vi "Intialize Sessions - 1Sess.vi"(6 "initialize and close session behavior":T1, 7 "option string":string, 8 "error in":errorcluster, 11 "session reservation in":refnum<class "Session Reservation.lvclass">) -> (0 "error out":errorcluster, 2 "session":refnum<class "Session Factory.lvclass">, 3 "session reservation out":refnum<class "Session Reservation.lvclass">)   [LabVIEW 2021, in "NI Session Management niSE.lvlib"]
uses:
  NI Session Management niSE.lvlib
  <vilib>/Plug-In SDKs/Clients/Session Management V1/Session Reservation/Session Reservation.lvclass
  <vilib>/Plug-In SDKs/Clients/Session Management V1/Session Reservation/Initialize and Close Session Behavior.ctl
  Session Factory/Session Factory.lvclass
  C:/Program Files/National Instruments/LabVIEW 2021/vi.lib/Plug-In SDKs/Sessions/Instrument/ISession Factory/ISession Factory.lvclass
  31e96d27-fcfd-4932-8456-b8131ef5f56a.vi
  <vilib>/Plug-In SDKs/Clients/Session Management V1/Session Reservation/Initialize Sessions with Retry.vi
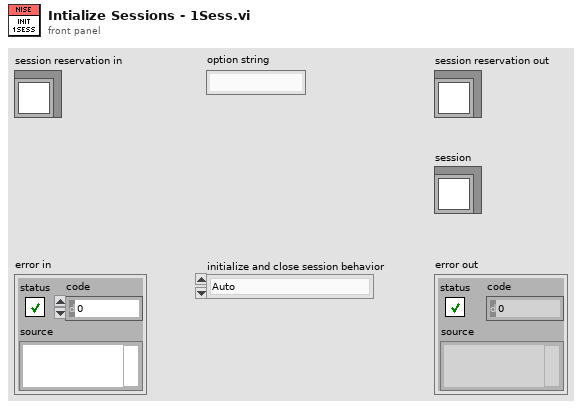
[diagram p1: front panel]
types:
  T1 = typedef "NI Session Management V1 Client.lvlib/Session Reservation.lvclass/Initialize and Close Session Behavior.ctl" = enum16{"Auto", "Initialize and Close", "Attach and Detach", "Initialize and Detach", "Attach and Close"}
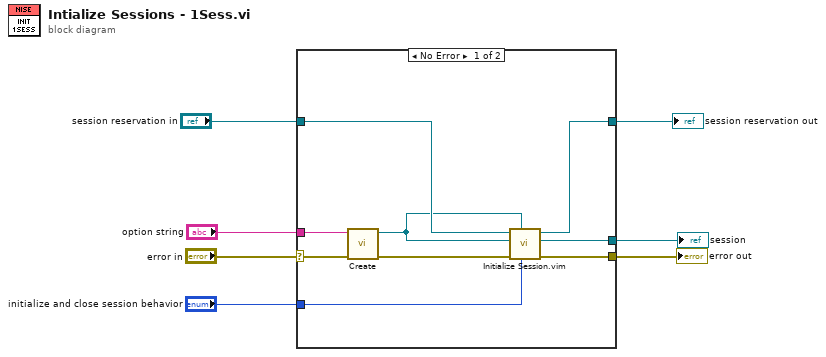
[diagram p0: block diagram]
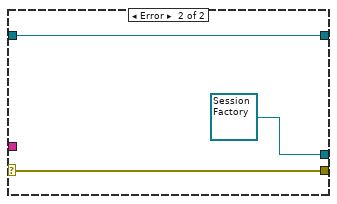
[diagram p2: hidden frame]
diagram:
  n1 = case shown="No Error" "error in" {
    selector: "error in" -> [w11 w18]
    tunnel: [w16 w18] -> w7
    tunnel: "initialize and close session behavior" -> [w15 _]
    tunnel: [w14 refnum<class "Session Factory.lvclass"> refnum ("session")] -> w1
    tunnel: [w13 w19] -> w5
    tunnel: "session reservation in" -> [w12 w19]
    tunnel: "option string" -> [w9 _]
    frame No Error {
      n2 = call "Create.vi"("error in (no error)"=w11, "Option String (\"\")"=w9) -> ("error out"=w10:errorcluster, "Session Factory out"=w8:refnum<class "Session Factory.lvclass">)  [unwired: 8 in]
      n3 = call "Initialize Session.vim"("initialize and close session behavior"=w15, "session type"=w8, "error in"=w10, "session factory"=w8, "session reservation in"=w12) -> ("error out"=w16:errorcluster, "session"=w14:refnum<class "Session Factory.lvclass">, "session reservation out"=w13:refnum<class "Session Reservation.lvclass">)  [unwired: 3 in, 1 out]
    }
    frame Error {
    }
  }
  "error out" <- w7
  "session reservation out" <- w5
  "session" <- w1
